vi "MIO Get QCurve.vi"(3 "Num Sweeps":i32=1) -> (0 "Waveform Graph":dbl[](graph))   [LabVIEW 2010]
uses:
  <vilib>/DAQmx/write.llb/DAQmx Write (Analog 1D DBL 1Chan NSamp).vi
  <vilib>/DAQmx/read.llb/DAQmx Read (Analog 1D DBL 1Chan NSamp).vi
  QCA Global.vi
  <vilib>/DAQmx/create/channels.llb/DAQmx Create Channel (AO-Voltage-Basic).vi
  <vilib>/DAQmx/configure/timing.llb/DAQmx Timing (Sample Clock).vi
  <vilib>/DAQmx/create/channels.llb/DAQmx Create Channel (CO-Pulse Generation-Time).vi
  <vilib>/DAQmx/configure/trigger.llb/DAQmx Start Trigger (Digital Edge).vi
  <vilib>/DAQmx/configure/timing.llb/DAQmx Timing (Implicit).vi
  <vilib>/DAQmx/create/channels.llb/DAQmx Create Channel (AI-Voltage-Basic).vi
  <vilib>/daqmx/miscellaneous.llb/DAQmx Fill In Error Info.vi
  Program Files (x86)/National Instruments/LabVIEW 2010/resource/objmgr/daqmx.rc
panel:
  in  "input terminal config":i32(ring)=-1 items=["default"=-1, "RSE"=10083, "NRSE"=10078, "Differential"=10106, "Pseudodifferential"=12529]
  out "Tune":dbl(slide) scale=-1.0..1.0 scale format="%.2f"
  out "Triangle Wave":dbl[](graph)=[-1.0, -0.996, -0.992, -0.988, -0.984, -0.98, -0.976, -0.972, -0.968, -0.964, -0.96, -0.956, -0.952, -0.948, -0.944, -0.94, -0.9359999999999999, -0.9319999999999999, -0.928, -0.924, -0.92, -0.916, -0.912, -0.908, -0.904, -0.9, -0.896, -0.892, -0.888, -0.884, -0.88, -0.876, -0.872, -0.868, -0.864, -0.86, -0.856, -0.852, -0.848, -0.844, -0.84, -0.836, -0.832, -0.8280000000000001, -0.8240000000000001, -0.8200000000000001, -0.8160000000000001, -0.812, -0.808, -0.804, -0.8, -0.796, -0.792, -0.788, -0.784, -0.78, -0.776, -0.772, -0.768, -0.764, -0.76, -0.756, -0.752, -0.748, -0.744, -0.74, -0.736, -0.732, -0.728, -0.724, -0.72, -0.716, -0.712, -0.708, -0.704, -0.7, -0.696, -0.692, -0.688, -0.6839999999999999, -0.6799999999999999, -0.6759999999999999, -0.6719999999999999, -0.6679999999999999, -0.6639999999999999, -0.6599999999999999, -0.656, -0.652, -0.648, -0.644, -0.64, -0.636, -0.632, -0.628, -0.624, -0.62, -0.616, -0.612, -0.608, -0.604, -0.6, -0.596, -0.5920000000000001, -0.5880000000000001, -0.5840000000000001, -0.5800000000000001, -0.5760000000000001, -0.5720000000000001, -0.5680000000000001, -0.5640000000000001, -0.56, -0.556, -0.552, -0.548, -0.544, -0.54, -0.536, -0.532, -0.528, -0.524, -0.52, -0.516, -0.512, -0.508, -0.504, -0.5, -0.496, -0.492, -0.488, -0.484, -0.48, -0.476, -0.472, -0.46799999999999997, -0.46399999999999997, -0.45999999999999996, -0.45599999999999996, -0.45199999999999996, -0.44799999999999995, -0.44399999999999995, -0.43999999999999995, -0.43600000000000005, -0.43200000000000005, -0.42800000000000005, -0.42400000000000004, -0.42000000000000004, -0.41600000000000004, -0.41200000000000003, -0.40800000000000003, -0.404, -0.4, -0.396, -0.392, -0.388, -0.384, -0.38, -0.376, -0.372, -0.368, -0.364, -0.36, -0.356, -0.352, -0.348, -0.344, -0.33999999999999997, -0.33599999999999997, -0.33199999999999996, -0.32799999999999996, -0.32399999999999995, -0.31999999999999995, -0.31599999999999995, -0.31200000000000006, -0.30800000000000005, -0.30400000000000005, -0.30000000000000004, -0.29600000000000004, -0.29200000000000004, -0.28800000000000003, -0.28400000000000003, -0.28, -0.276, -0.272, -0.268, -0.264, -0.26, -0.256, -0.252, -0.248, -0.244, -0.24, -0.236, -0.23199999999999998, -0.22799999999999998, -0.22399999999999998, -0.21999999999999997, -0.21599999999999997, -0.21199999999999997, -0.20799999999999996, -0.20399999999999996, -0.19999999999999996, -0.19599999999999995, -0.19199999999999995, -0.18799999999999994, -0.18400000000000005, -0.18000000000000005, -0.17600000000000005, -0.17200000000000004, -0.16800000000000004, -0.16400000000000003, -0.16000000000000003, -0.15600000000000003, -0.15200000000000002, -0.14800000000000002, -0.14400000000000002, -0.14, -0.136, -0.132, -0.128, -0.124, -0.12, -0.11599999999999999, -0.11199999999999999, -0.10799999999999998, -0.10399999999999998, -0.09999999999999998, -0.09599999999999997, -0.09199999999999997, -0.08799999999999997, -0.08399999999999996, -0.07999999999999996, -0.07599999999999996, -0.07199999999999995, -0.06799999999999995, -0.06399999999999995, -0.06000000000000005, -0.05600000000000005, -0.052000000000000046, -0.04800000000000004, -0.04400000000000004, -0.040000000000000036, -0.03600000000000003, -0.03200000000000003, -0.028000000000000025, -0.02400000000000002, -0.020000000000000018, -0.016000000000000014, -0.01200000000000001, -0.008000000000000007, -0.0040000000000000036, 0.0, 0.0040000000000000036, 0.008000000000000007, 0.01200000000000001, 0.016000000000000014, 0.020000000000000018, 0.02400000000000002, 0.028000000000000025, 0.03200000000000003, 0.03600000000000003, 0.040000000000000036, 0.04400000000000004, 0.04800000000000004, 0.052000000000000046, 0.05600000000000005, 0.06000000000000005, 0.06400000000000006, 0.06800000000000006, 0.07200000000000006, 0.07600000000000007, 0.08000000000000007, 0.08400000000000007, 0.08800000000000008, 0.09200000000000008, 0.09600000000000009, 0.10000000000000009, 0.10400000000000009, 0.1080000000000001, 0.1120000000000001, 0.1160000000000001, 0.1200000000000001, 0.12400000000000011, 0.1279999999999999, 0.1319999999999999, 0.1359999999999999, 0.1399999999999999, 0.1439999999999999, 0.1479999999999999, 0.1519999999999999, 0.15599999999999992, 0.15999999999999992, 0.16399999999999992, 0.16799999999999993, 0.17199999999999993, 0.17599999999999993, 0.17999999999999994, 0.18399999999999994, 0.18799999999999994, 0.19199999999999995, 0.19599999999999995, 0.19999999999999996, 0.20399999999999996, 0.20799999999999996, 0.21199999999999997, 0.21599999999999997, 0.21999999999999997, 0.22399999999999998, 0.22799999999999998, 0.23199999999999998, 0.236, 0.24, 0.244, 0.248, 0.252, 0.256, 0.26, 0.264, 0.268, 0.272, 0.276, 0.28, 0.28400000000000003, 0.28800000000000003, 0.29200000000000004, 0.29600000000000004, 0.30000000000000004, 0.30400000000000005, 0.30800000000000005, 0.31200000000000006, 0.31600000000000006, 0.32000000000000006, 0.32400000000000007, 0.32800000000000007, 0.3320000000000001, 0.3360000000000001, 0.3400000000000001, 0.3440000000000001, 0.3480000000000001, 0.3520000000000001, 0.3560000000000001, 0.3600000000000001, 0.3640000000000001, 0.3680000000000001, 0.3720000000000001, 0.3759999999999999, 0.3799999999999999, 0.3839999999999999, 0.3879999999999999, 0.3919999999999999, 0.3959999999999999, 0.3999999999999999, 0.4039999999999999, 0.4079999999999999, 0.4119999999999999, 0.4159999999999999, 0.41999999999999993, 0.42399999999999993, 0.42799999999999994, 0.43199999999999994, 0.43599999999999994, 0.43999999999999995, 0.44399999999999995, 0.44799999999999995, 0.45199999999999996, 0.45599999999999996, 0.45999999999999996, 0.46399999999999997, 0.46799999999999997, 0.472, 0.476, 0.48, 0.484, 0.488, 0.492, 0.496, 0.5, 0.504, 0.508, 0.512, 0.516, 0.52, 0.524, 0.528, 0.532, 0.536, 0.54, 0.544, 0.548, 0.552, 0.556, 0.56, 0.5640000000000001, 0.5680000000000001, 0.5720000000000001, 0.5760000000000001, 0.5800000000000001, 0.5840000000000001, 0.5880000000000001, 0.5920000000000001, 0.5960000000000001, 0.6000000000000001, 0.6040000000000001, 0.6080000000000001, 0.6120000000000001, 0.6160000000000001, 0.6200000000000001, 0.6240000000000001, 0.6279999999999999, 0.6319999999999999, 0.6359999999999999, 0.6399999999999999, 0.6439999999999999, 0.6479999999999999, 0.6519999999999999, 0.6559999999999999, 0.6599999999999999, 0.6639999999999999, 0.6679999999999999, 0.6719999999999999, 0.6759999999999999, 0.6799999999999999, 0.6839999999999999, 0.688, 0.692, 0.696, 0.7, 0.704, 0.708, 0.712, 0.716, 0.72, 0.724, 0.728, 0.732, 0.736, 0.74, 0.744, 0.748, 0.752, 0.756, 0.76, 0.764, 0.768, 0.772, 0.776, 0.78, 0.784, 0.788, 0.792, 0.796, 0.8, 0.804, 0.808, 0.812, 0.8160000000000001, 0.8200000000000001, 0.8240000000000001, 0.8280000000000001, 0.8320000000000001, 0.8360000000000001, 0.8400000000000001, 0.8440000000000001, 0.8480000000000001, 0.8520000000000001, 0.8560000000000001, 0.8600000000000001, 0.8640000000000001, 0.8680000000000001, 0.8720000000000001, 0.8759999999999999, 0.8799999999999999, 0.8839999999999999, 0.8879999999999999, 0.8919999999999999, 0.8959999999999999, 0.8999999999999999, 0.9039999999999999, 0.9079999999999999, 0.9119999999999999, 0.9159999999999999, 0.9199999999999999, 0.9239999999999999, 0.9279999999999999, 0.9319999999999999, 0.9359999999999999, 0.94, 0.944, 0.948, 0.952, 0.956, 0.96, 0.964, 0.968, 0.972, 0.976, 0.98, 0.984, 0.988, 0.992, 0.996]
  # "A\nD\nD\n\nP\nH\nA\nS\nE"
  # "R\nE\nM\nO\nV\nE\n\nP\nH\nA\nS\nE"
  # "A\nD\nD\n\nP\nH\nA\nS\nE"
  # "R\nE\nM\nO\nV\nE\n\nP\nH\nA\nS\nE"
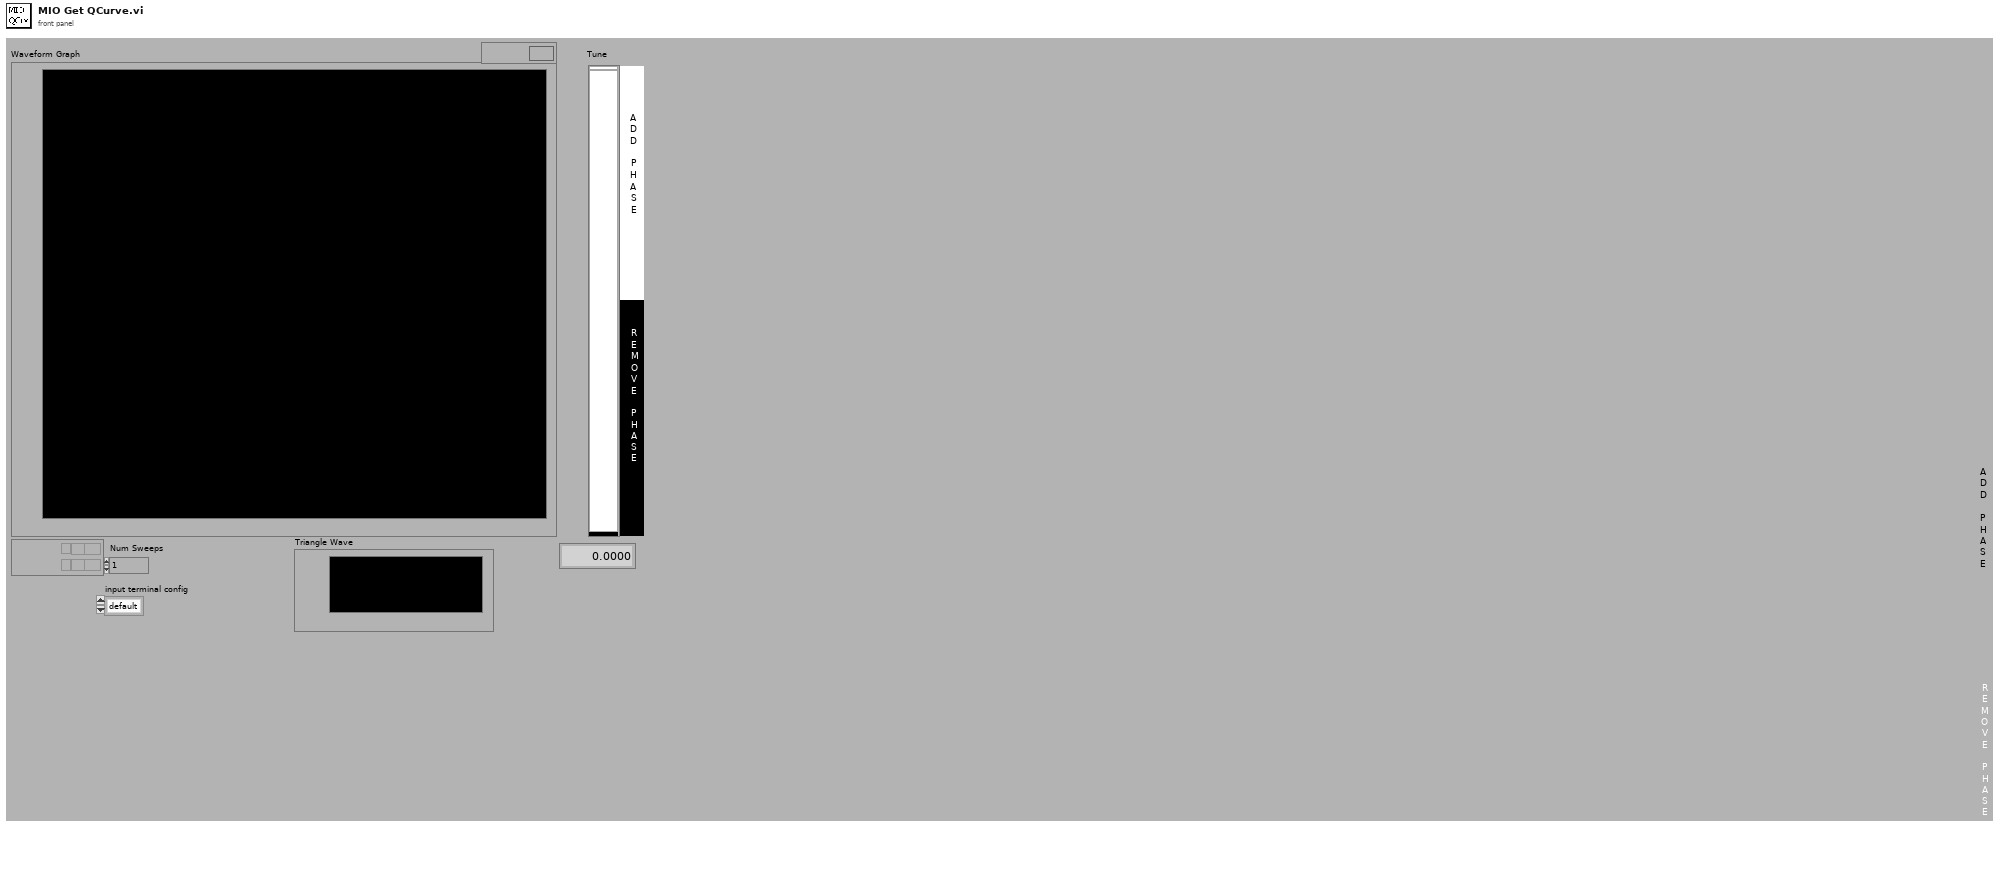
[diagram p1: front panel]
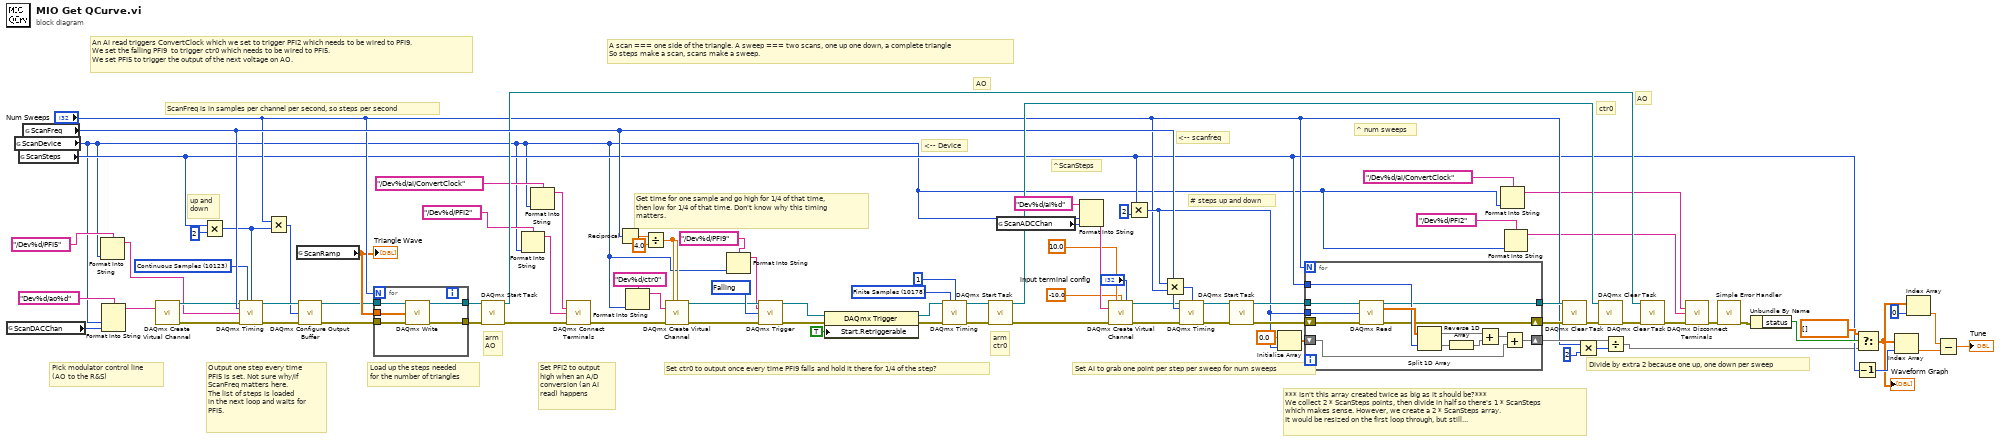
[diagram p0: block diagram]
diagram:
  w36 = 10171 items=["Rising"=10280, "Falling"=10171] ("edge")
  w51 = 10123 items=["Finite Samples"=10178, "Continuous Samples"=10123, "Hardware Timed Single Point"=12522] ("sample mode")
  w83 = 10178 items=["Finite Samples"=10178, "Continuous Samples"=10123, "Hardware Timed Single Point"=12522] ("sample mode")
  # "Divide by extra 2 because one up, one down per sweep"
  # "*** Isn't this array created twice as big as it should be?***\nWe collect 2 * ScanSteps points, then divide in half so there's 1 * ScanSteps\nwhich makes sense. However, we create a 2 * ScanSteps array.\nIt would be resized on the first loop through, but still..."
  # "# steps up and down"
  # "^ScanSteps"
  # "Get time for one sample and go high for 1/4 of that time,\nthen low for 1/4 of that time. Don't know why this timing\nmatters."
  # "A scan === one side of the triangle. A sweep === two scans, one up one down, a complete triangle\nSo steps make a scan, scans make a sweep."
  # "up and\ndown"
  # "ScanFreq is in samples per channel per second, so steps per second"
  # "<-- Device"
  # "<-- scanfreq"
  # "ctr0"
  # "AO"
  # "arm\nctr0"
  # "An AI read triggers ConvertClock which we set to trigger PFI2 which needs to be wired to PFI9.\nWe set the falling PFI9  to trigger ctr0 which needs to be wired to PFI5.\nWe set PFI5 to trigger the output of the next voltage on AO."
  # "arm\nAO"
  # "Load up the steps needed\nfor the number of triangles"
  # "AO"
  # "^ num sweeps"
  # "Set PFI2 to output\nhigh when an A/D\nconversion (an AI\nread) happens"
  # "Output one step every time\nPFI5 is set. Not sure why/if\nScanFreq matters here.\nThe list of steps is loaded\nin the next loop and waits for\nPFI5."
  # "Set AI to grab one point per step per sweep for num sweeps"
  # "Set ctr0 to output once every time PFI9 falls and hold it there for 1/4 of the step?"
  # "Pick modulator control line\n(AO to the R&S)"
  n1 = global read "QCA Global.vi" "ScanDACChan"() -> (w26:i32)
  n2 = global read "QCA Global.vi" "ScanDevice"() -> (w4:i32)
  n3 = global read "QCA Global.vi" "ScanSteps"() -> (w19:i32)
  n4 = global read "QCA Global.vi" "ScanFreq"() -> (w89:i32)
  n5 = Format Into String(format string="/Dev%d/PFI5", w4) -> (resulting string=w14:string)  [unwired: 2 in, 1 out]
  n6 = Format Into String(format string="Dev%d/ao%d", w4, w26) -> (resulting string=w27:string)  [unwired: 2 in, 1 out]
  n7 = call-poly <vilib>:"DAQmx Create Virtual Channel.vi"("physical channels"=w27) -> ("task out"=w39:refnum<k21>, "error out"=w38:errorcluster)  [unwired: 13 in]
  n8 = Multiply(x=w19, y=2) -> (x*y=w47:i32)
  n9 = call-poly <vilib>:"DAQmx Timing.vi"("task/channels in"=w39, "sample mode"=w51, "samples per channel"=w47, "rate"=w89, "source"=w14, "error in"=w38) -> ("task out"=w49:refnum<k21>, "error out"=w48:errorcluster)  [unwired: 8 in]
  n10 = Multiply(x="Num Sweeps", y=w47) -> (x*y=w45:i32)
  n11 = global read "QCA Global.vi" "ScanRamp"() -> (w44:dbl[])
  "Triangle Wave" <- w44
  n12 = call <vilib>:"DAQmx Configure Output Buffer.vi"("task/channels in"=w49, "buffer size (in samples per channel)"=w45, "error in"=w48) -> ("task out"=w42:refnum<k21>, "error out"=w43:errorcluster)  [unwired: 11 in]
  n13 = for {
    N: "Num Sweeps" -> [_]
    tunnel: w44 -> [w95]
    tunnel: w43 -> [w94]
    tunnel: w42 -> [w93]
    tunnel: [w92] -> w41
    tunnel: [w91] -> w40
    n14 = call-poly <vilib>:"DAQmx Write.vi"("task/channels in"=w93, "data"=w95, "error in"=w94) -> ("task out"=w92:refnum<k21>, "error out"=w91:errorcluster)  [unwired: 10 in, 1 out]
  }
  n15 = call <vilib>:"DAQmx Start Task.vi"("task/channels in"=w41, "error in"=w40) -> ("task out"=w50:refnum<k21>, "error out"=w88:errorcluster)  [unwired: 12 in]
  n16 = Format Into String(format string="/Dev%d/PFI2", w4) -> (resulting string=w10:string)  [unwired: 2 in, 1 out]
  n17 = Format Into String(format string="/Dev%d/ai/ConvertClock", w4) -> (resulting string=w13:string)  [unwired: 2 in, 1 out]
  n18 = call <vilib>:"DAQmx Connect Terminals.vi"("source terminal"=w13, "destination terminal"=w10, "error in"=w88) -> ("error out"=w87:errorcluster)  [unwired: 12 in]
  n19 = Reciprocal(x=w89) -> (1/x=w85:dbl)
  n20 = Format Into String(format string="Dev%d/ctr0", w4) -> (resulting string=w21:string)  [unwired: 2 in, 1 out]
  n21 = Divide(x=w85, y=4.0) -> (x/y=w84:dbl)
  n22 = call-poly <vilib>:"DAQmx Create Virtual Channel.vi"("high time"=w84, "low time"=w84, "counter"=w21, "error in"=w87) -> ("task out"=w35:refnum<k21>, "error out"=w37:errorcluster)  [unwired: 10 in]
  n23 = Format Into String(format string="/Dev%d/PFI9", w4) -> (resulting string=w8:string)  [unwired: 2 in, 1 out]
  n24 = call-poly <vilib>:"DAQmx Trigger.vi"("task/channels in"=w35, "source"=w8, "edge"=w36, "error in"=w37) -> ("task out"=w33:refnum<k21>, "error out"=w32:errorcluster)  [unwired: 10 in]
  n25 = property class="DAQmx Trigger"(reference=w33, error in=w32, "Start.Retriggerable"=TRUE) -> (reference out=w31:refnum<k21>, error out=w30:errorcluster)
  n26 = call-poly <vilib>:"DAQmx Timing.vi"("task/channels in"=w31, "sample mode"=w83, "samples per channel"=1, "error in"=w30) -> ("task out"=w82:refnum<k21>, "error out"=w81:errorcluster)  [unwired: 10 in]
  n27 = call <vilib>:"DAQmx Start Task.vi"("task/channels in"=w82, "error in"=w81) -> ("task out"=w90:refnum<k21>, "error out"=w80:errorcluster)  [unwired: 12 in]
  n28 = global read "QCA Global.vi" "ScanADCChan"() -> (w24:i32)
  n29 = Format Into String(format string="Dev%d/ai%d", w4, w24) -> (resulting string=w23:string)  [unwired: 2 in, 1 out]
  n30 = call-poly <vilib>:"DAQmx Create Virtual Channel.vi"("maximum value"=10.0, "minimum value"=-10.0, "input terminal configuration"="input terminal config", "physical channels"=w23, "error in"=w80) -> ("task out"=w79:refnum<k21>, "error out"=w78:errorcluster)  [unwired: 9 in]
  n31 = Multiply(x=w19, y=2) -> (x*y=w53:i32)
  n32 = Multiply(x=w53, y="Num Sweeps") -> (x*y=w77:i32)
  n33 = call-poly <vilib>:"DAQmx Timing.vi"("task/channels in"=w79, "samples per channel"=w77, "rate"=w89, "error in"=w78) -> ("task out"=w76:refnum<k21>, "error out"=w75:errorcluster)  [unwired: 10 in]
  n34 = call <vilib>:"DAQmx Start Task.vi"("task/channels in"=w76, "error in"=w75) -> ("task out"=w70:refnum<k21>, "error out"=w74:errorcluster)  [unwired: 12 in]
  n35 = Initialize Array(sgl 0.0 ("Element Data"), w53) -> (w71:sgl[])
  n36 = for {
    N: "Num Sweeps" -> [_]
    shift-right: [w98] -> w67
    shift-left: w74 -> [w96]
    shift-right: [w101] -> w69
    shift-left: w71 -> [w99]
    tunnel: w70 -> [w108]
    tunnel: w53 -> [w107]
    tunnel: w19 -> [w105]
    tunnel: [w97] -> w68
    n37 = call-poly <vilib>:"DAQmx Read.vi"("task/channels in"=w108, "number of samples per channel"=w107, "error in"=w96) -> ("task out"=w97:refnum<k21>, "data"=w106:dbl[], "error out"=w98:errorcluster)  [unwired: 10 in]
    n38 = Split 1D Array(array=w106, index=w105) -> (first subarray=w103:dbl[], second subarray=w104:dbl[])
    n39 = Reverse 1D Array(array=w104) -> (reversed array=w102:dbl[])
    n40 = Add(x=w103, y=w102) -> (x+y=w100:dbl[])
    n41 = Add(x=w100, y=w99) -> (x+y=w101:dbl[])
  }
  n42 = Format Into String(format string="/Dev%d/ai/ConvertClock", w4) -> (resulting string=w6:string)  [unwired: 2 in, 1 out]
  n43 = Format Into String(format string="/Dev%d/PFI2", w4) -> (resulting string=w3:string)  [unwired: 2 in, 1 out]
  n44 = call <vilib>:"DAQmx Clear Task.vi"("task in"=w68, "error in"=w67) -> ("error out"=w66:errorcluster)  [unwired: 13 in]
  n45 = Multiply(x="Num Sweeps", y=2) -> (x*y=w17:i32)
  n46 = call <vilib>:"DAQmx Clear Task.vi"("task in"=w90, "error in"=w66) -> ("error out"=w65:errorcluster)  [unwired: 13 in]
  n47 = Divide(x=w69, y=w17) -> (x/y=w18:dbl[])
  n48 = call <vilib>:"DAQmx Clear Task.vi"("task in"=w50, "error in"=w65) -> ("error out"=w55:errorcluster)  [unwired: 13 in]
  n49 = call <vilib>:"DAQmx Disconnect Terminals.vi"("source terminal"=w6, "destination terminal"=w3, "error in"=w55) -> ("error out"=w54:errorcluster)  [unwired: 12 in]
  n50 = call <vilib>:"Simple Error Handler.vi"("error in (no error)"=w54) -> ("error out"=w64:errorcluster)  [unwired: 4 in, 4 out]
  n51 = Unbundle By Name(w64) -> ("status"=w62:bool)
  n52 = Decrement(x=w19) -> (x-1=w58:i32)
  n53 = Select(t=dbl[] [], s=w62, f=w18) -> (s? t:f=w56:dbl[])
  "Waveform Graph" <- w56
  n54 = Index Array(array=w56, index=w58) -> (element=w61:dbl)
  n55 = Index Array(array=w56, index=0 ("Index")) -> (element=w60:dbl)
  n56 = Subtract(x=w60, y=w61) -> (x-y=→"Tune":dbl)
